vi "Image Mask.vi"() -> ()   [LabVIEW 2014]
doc: "This example shows how to apply a mask to another image. The mask is a binary image.\n\nFor each pixel in the mask that has a value of zero, the corresponding pixel in the original image will be set to zero in the output image, <B>Masked Image</B>. All other pixels in the output will retain the same values from the original image.\n\nMasking is an effective way to process specific parts of an image."
uses:
  <vilib>/vision/NI_Vision_Development_Module.lvlib
panel:
  in  "Rotated Rectangle Coordinates":T1={"Left"=20, "Top"=20, "Right"=100, "Bottom"=75, "Rotation"=40.0} {"Rotation" format="%.2f"; "Left" scale=0.0..1024.0; "Right" scale=0.0..1024.0}
  out "Masked Image":T2(plugin-control)
  out "Mask Image":T2(plugin-control)
  out "Image Source":T2(plugin-control)
  in  "Y Offset":i32=60
  in  "X Offset":i32=85
  # "Overview: Demonstrates how to build an image mask and use it to mask out a portion of an image.\nRequirements: NI Vision Development Module\nInstructions: Run the VI."
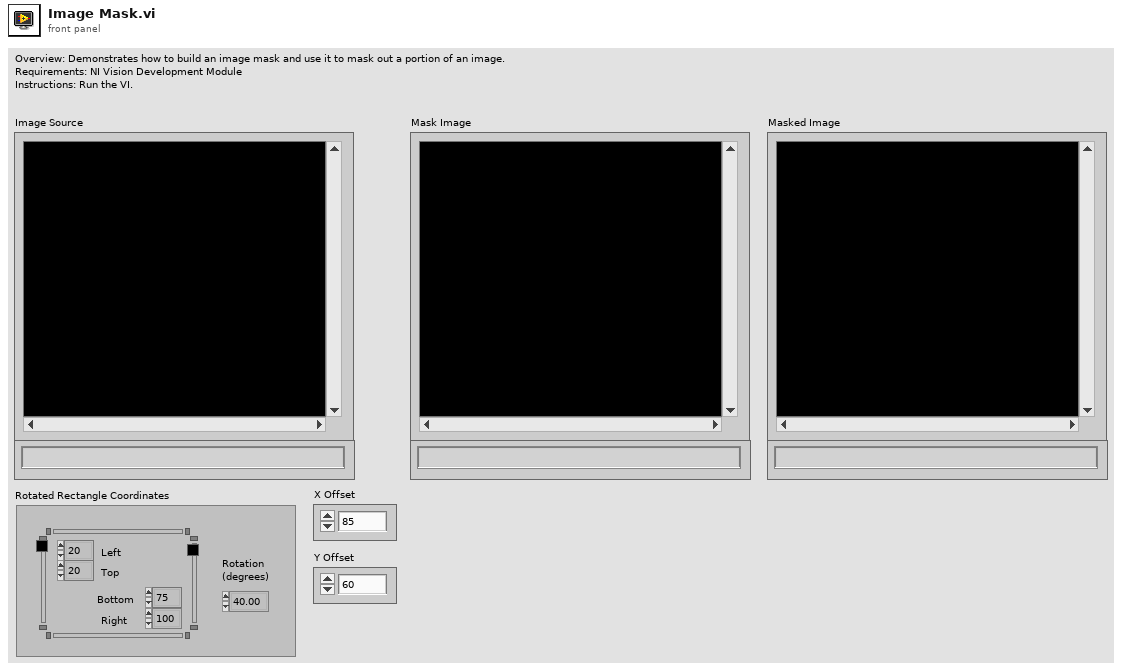
[diagram p1: front panel]
types:
  T1 = typedef "IMAQ Rectangle" = cluster{"Left":i32, "Top":i32, "Right":i32, "Bottom":i32, "Rotation":dbl}
  T2 = typedef "IMAQ Image.ctl" = refnum<image>
  T3 = typedef "Image Type" = u32
  T4 = typedef "ROI Descriptor" = cluster{"Global Rectangle":i32[], "Contours":cluster{"ID":enum32{"External", "Internal"}, "Type":u32, "Coordinates":i32[]}[]}
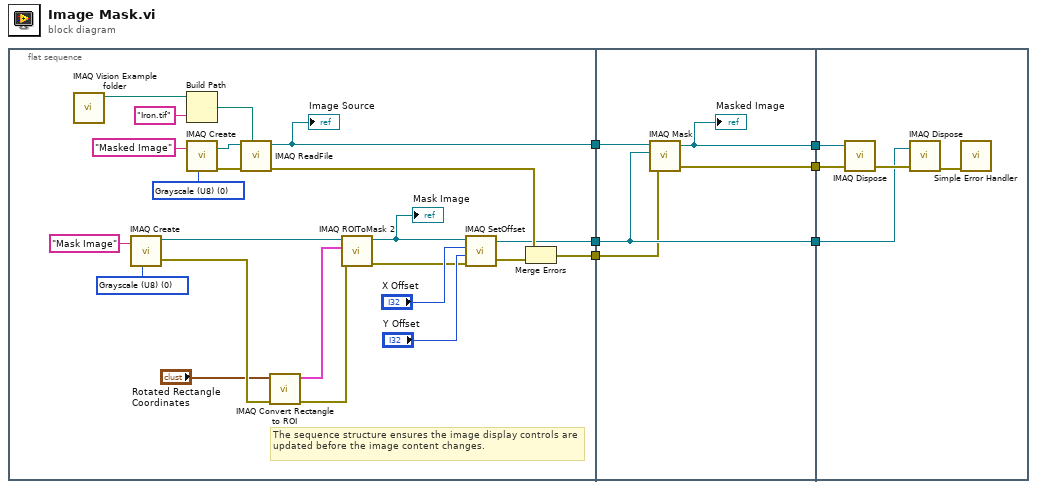
[diagram p0: block diagram]
diagram:
  n1 = flat-sequence {
    tunnel: [w8] -> w6
    tunnel: [w16] -> w2
    tunnel: [w15] -> w1
    tunnel: w6 -> [w34]
    tunnel: [w33] -> w5
    tunnel: [w32] -> w4
    tunnel: [w31] -> w3
    tunnel: w2 -> [w31]
    tunnel: w1 -> [w30]
    tunnel: w5 -> [w37]
    tunnel: w4 -> [w36]
    tunnel: w3 -> [w35]
    frame #0 {
      w22 = T3 0 items=["Grayscale (U8)", "Grayscale (I16)", "Grayscale (SGL)", "Complex (CSG)", "RGB (U32)", "HSL (U32)", "RGB (U64)", "Grayscale (U16)"] ("Image Type")
      w23 = T3 0 items=["Grayscale (U8)", "Grayscale (I16)", "Grayscale (SGL)", "Complex (CSG)", "RGB (U32)", "HSL (U32)", "RGB (U64)", "Grayscale (U16)"] ("Image Type")
      # "The sequence structure ensures the image display controls are updated before the image content changes."
      n2 = call "IMAQ Vision Example folder.vi"() -> ("Example Image Path"=w21:path)  [unwired: 11 in]
      n3 = call "IMAQ Create"("Image Name"="Mask Image", "Image Type"=w22) -> ("New Image"=w14:T2, "error out"=w11:errorcluster)  [unwired: 3 in]
      n4 = Build Path(base path=w21, name or relative path="Iron.tif") -> (appended path=w24:path)
      n5 = call "IMAQ Create"("Image Name"="Masked Image", "Image Type"=w23) -> ("New Image"=w26:T2, "error out"=w25:errorcluster)  [unwired: 3 in]
      n6 = call "IMAQ ReadFile"("File Path"=w24, "error in (no error)"=w25, "Image"=w26) -> ("error out"=w20:errorcluster, "Image Out"=w8:T2)  [unwired: 4 in, 3 out]
      "Image Source" <- w8
      n7 = call "IMAQ Convert Rectangle to ROI"("error in (no error)"=w11, "Rectangle"="Rotated Rectangle Coordinates") -> ("error out"=w10:errorcluster, "ROI Descriptor"=w9:T4)  [unwired: 7 in]
      n8 = call "IMAQ ROIToMask 2"("error in (no error)"=w10, "ROI Descriptor"=w9, "Image"=w14) -> ("error out"=w12:errorcluster, "Image Out"=w13:T2)  [unwired: 6 in, 1 out]
      "Mask Image" <- w13
      n9 = call "IMAQ SetOffset"("error in (no error)"=w12, "Y Offset"="Y Offset", "X Offset"="X Offset", "Image"=w13) -> ("error out"=w17:errorcluster, "Image Out"=w16:T2)
      n10 = Merge Errors(w20, w17) -> (w15:errorcluster)
    }
    frame #1 {
      n11 = call "IMAQ Mask"("error in (no error)"=w30, "Image Mask"=w31, "Image Src"=w34) -> ("error out"=w32:errorcluster, "Image Dst Out"=w33:T2)  [unwired: 2 in]
      "Masked Image" <- w33
    }
    frame #2 {
      n12 = call "IMAQ Dispose"("Image"=w37, "error in (no error)"=w36) -> ("error out"=w38:errorcluster)  [unwired: 4 in]
      n13 = call "IMAQ Dispose"("Image"=w35, "error in (no error)"=w38) -> ("error out"=w39:errorcluster)  [unwired: 4 in]
      n14 = call <vilib>:"Simple Error Handler.vi"("error in (no error)"=w39) -> ()  [unwired: 4 in, 5 out]
    }
  }
